vi "shortDescription.vi"(8 "error in (no error)":errorcluster, 11 "TestCase in":refnum<class "TestCase.lvclass">) -> (0 "error out":errorcluster, 2 "description":string, 3 "TestCase out":refnum<class "TestCase.lvclass">)   [LabVIEW 2013, in "TestCase.lvclass"]
uses:
  TestCase.lvclass
  TestCase.lvclass/TestCase.ctl
  <userlib>/_OpenG.lib/string/string.llb/Trim Whitespace (String)__ogtk.vi
panel:
  # "JKI VI Tester for LabVIEW\nhttp://jkisoft.com/vi-tester\nCopyright (C) 2007-2009, JKI <info@jkisoft.com>\nALL RIGHTS RESERVED"
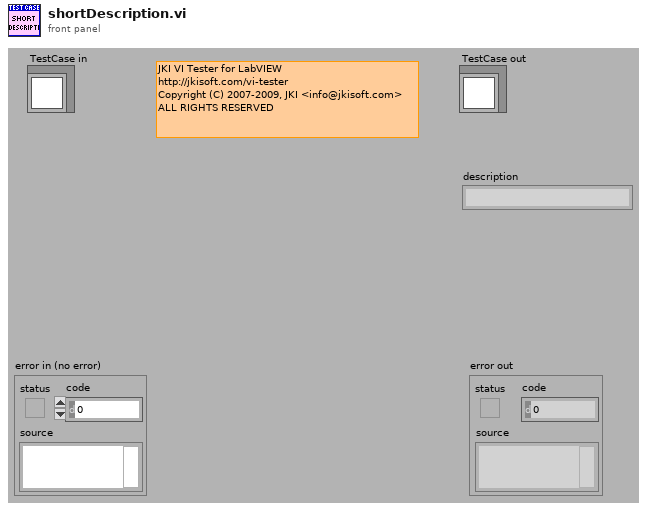
[diagram p1: front panel]
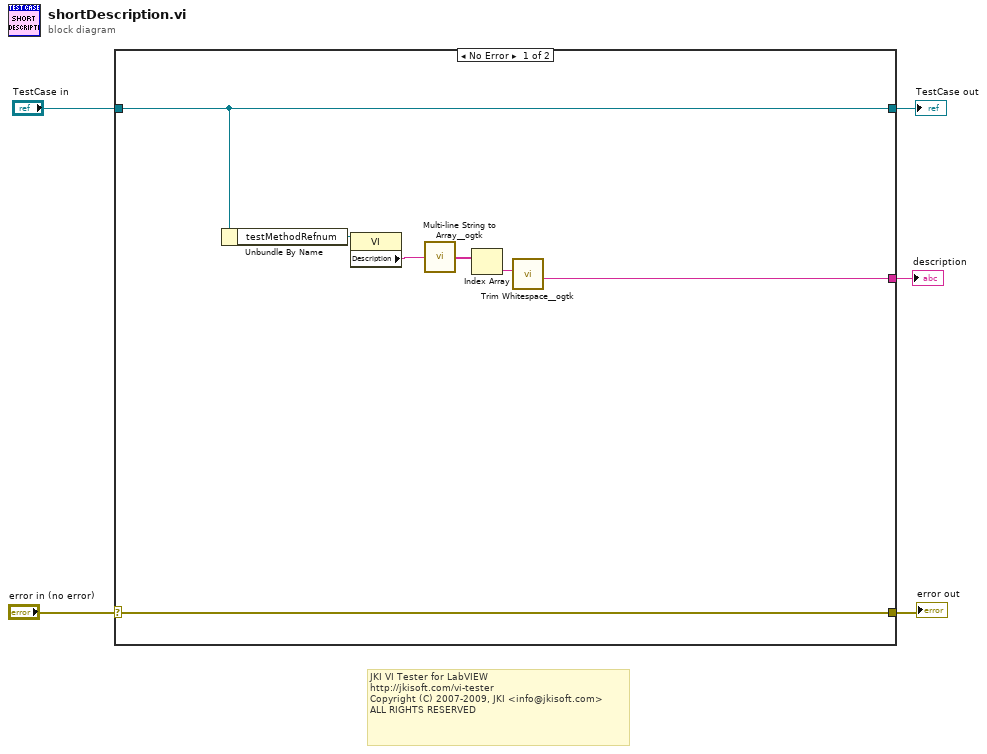
[diagram p0: block diagram]
diagram:
  # "JKI VI Tester for LabVIEW\nhttp://jkisoft.com/vi-tester\nCopyright (C) 2007-2009, JKI <info@jkisoft.com>\nALL RIGHTS RESERVED"
  n1 = case shown="No Error" "error in (no error)" {
    selector: "error in (no error)" -> [w12 w14]
    tunnel: [w12 w14] -> w4
    tunnel: [w11 w13] -> w2
    tunnel: "TestCase in" -> [w11 w13]
    tunnel: [w6 _] -> w1
    frame No Error {
      n2 = Unbundle By Name(w11) -> ("testMethodRefnum"=w10:refnum<vi>)
      n3 = property class="VI"(reference=w10) -> ("Description"=w9:string)  [unwired: 1 in, 2 out]
      n4 = call <userlib>:"Multi-line String to Array__ogtk.vi"("string"=w9) -> ("lines"=w8:string[])
      n5 = Index Array(array=w8) -> (element=w7:string)  [unwired: 1 in]
      n6 = call-poly <userlib>:"Trim Whitespace__ogtk.vi"("String in"=w7) -> ("String out"=w6:string)  [unwired: 6 in]
    }
    frame Error {
    }
  }
  "error out" <- w4
  "TestCase out" <- w2
  "description" <- w1
